vi "Fader toScreen400.vi"(11 "Numeric":dbl) -> (3 "Numeric 2":dbl)   [LabVIEW 2011]
panel:
  out "x-y":dbl
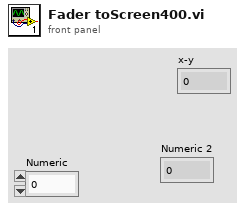
[diagram p1: front panel]
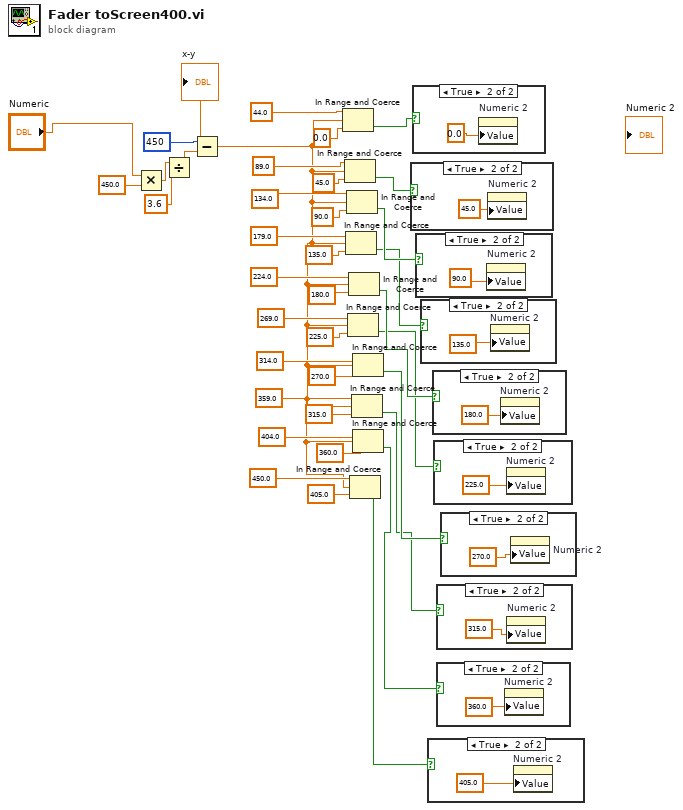
[diagram p0: block diagram]
diagram:
  n1 = Multiply(x="Numeric", y=450.0) -> (x*y=w36:dbl)
  n2 = Divide(x=w36, y=3.6) -> (x/y=w33:dbl)
  n3 = Subtract(x=450, y=w33) -> (x-y=w3:dbl)
  "x-y" <- w3
  n4 = In Range and Coerce(upper limit=44.0 ("lower limit"), x=w3, lower limit=0.0 ("upper limit")) -> (In Range?=w31:bool)  [unwired: 1 out]
  n5 = In Range and Coerce(upper limit=89.0 ("lower limit"), x=w3, lower limit=45.0 ("upper limit")) -> (In Range?=w30:bool)  [unwired: 1 out]
  n6 = In Range and Coerce(upper limit=179.0 ("lower limit"), x=w3, lower limit=135.0 ("upper limit")) -> (In Range?=w28:bool)  [unwired: 1 out]
  n7 = In Range and Coerce(upper limit=134.0 ("lower limit"), x=w3, lower limit=90.0 ("upper limit")) -> (In Range?=w29:bool)  [unwired: 1 out]
  n8 = In Range and Coerce(upper limit=269.0 ("lower limit"), x=w3, lower limit=225.0 ("upper limit")) -> (In Range?=w26:bool)  [unwired: 1 out]
  n9 = In Range and Coerce(upper limit=224.0 ("lower limit"), x=w3, lower limit=180.0 ("upper limit")) -> (In Range?=w27:bool)  [unwired: 1 out]
  n10 = In Range and Coerce(upper limit=450.0 ("lower limit"), x=w3, lower limit=405.0 ("upper limit")) -> (In Range?=w1:bool)  [unwired: 1 out]
  n11 = In Range and Coerce(upper limit=359.0 ("lower limit"), x=w3, lower limit=315.0 ("upper limit")) -> (In Range?=w24:bool)  [unwired: 1 out]
  n12 = In Range and Coerce(upper limit=314.0 ("lower limit"), x=w3, lower limit=270.0 ("x")) -> (In Range?=w25:bool)  [unwired: 1 out]
  n13 = In Range and Coerce(upper limit=404.0 ("lower limit"), x=w3, lower limit=360.0 ("upper limit")) -> (In Range?=w2:bool)  [unwired: 1 out]
  n14 = case shown="True" w30 {
    frame False {
    }
    frame True {
      n15 = property on="Numeric 2" class="DigNum (strict)"("Value"=45.0 ("Numeric 2")) -> ()  [unwired: 2 in, 2 out]
    }
  }
  n16 = case shown="True" w31 {
    frame False {
    }
    frame True {
      n17 = property on="Numeric 2" class="DigNum (strict)"("Value"=0.0 ("Numeric 2")) -> ()  [unwired: 2 in, 2 out]
    }
  }
  n18 = case shown="True" w29 {
    frame False {
    }
    frame True {
      n19 = property on="Numeric 2" class="DigNum (strict)"("Value"=90.0 ("Numeric 2")) -> ()  [unwired: 2 in, 2 out]
    }
  }
  n20 = case shown="True" w28 {
    frame False {
    }
    frame True {
      n21 = property on="Numeric 2" class="DigNum (strict)"("Value"=135.0 ("Numeric 2")) -> ()  [unwired: 2 in, 2 out]
    }
  }
  n22 = case shown="True" w1 {
    frame False {
    }
    frame True {
      n23 = property on="Numeric 2" class="DigNum (strict)"("Value"=405.0 ("Numeric 2")) -> ()  [unwired: 2 in, 2 out]
    }
  }
  n24 = case shown="True" w27 {
    frame False {
    }
    frame True {
      n25 = property on="Numeric 2" class="DigNum (strict)"("Value"=180.0 ("Numeric 2")) -> ()  [unwired: 2 in, 2 out]
    }
  }
  n26 = case shown="True" w26 {
    frame False {
    }
    frame True {
      n27 = property on="Numeric 2" class="DigNum (strict)"("Value"=225.0 ("Numeric 2")) -> ()  [unwired: 2 in, 2 out]
    }
  }
  n28 = case shown="True" w24 {
    frame False {
    }
    frame True {
      n29 = property on="Numeric 2" class="DigNum (strict)"("Value"=315.0 ("Numeric 2")) -> ()  [unwired: 2 in, 2 out]
    }
  }
  n30 = case shown="True" w2 {
    frame False {
    }
    frame True {
      n31 = property on="Numeric 2" class="DigNum (strict)"("Value"=360.0 ("Numeric 2")) -> ()  [unwired: 2 in, 2 out]
    }
  }
  n32 = case shown="True" w25 {
    frame False {
    }
    frame True {
      n33 = property on="Numeric 2" class="DigNum (strict)"("Value"=270.0 ("Numeric 2")) -> ()  [unwired: 2 in, 2 out]
    }
  }
